vi "E2E Save Instrument.vi"() -> ()   [LabVIEW 2026]
panel:
  out "error out":errorcluster
  in  "vi path":path
  in  "Path to Saved File":path
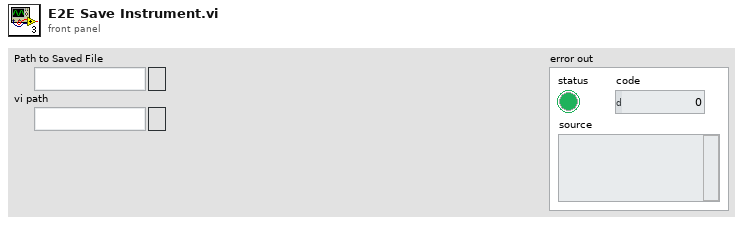
[diagram p1: front panel]
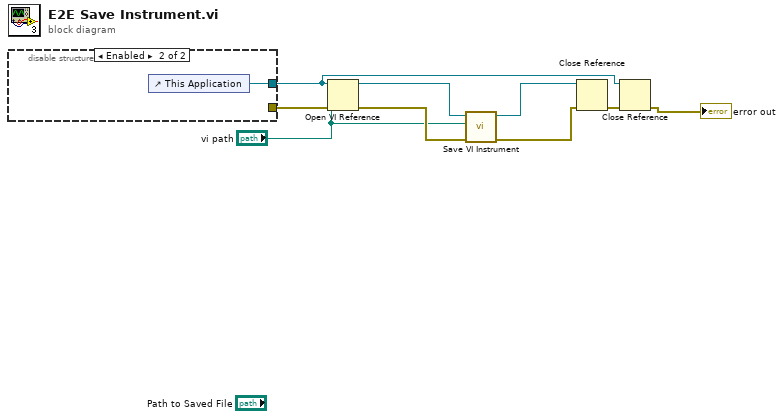
[diagram p0: block diagram]
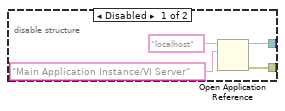
[diagram p2: hidden frame]
diagram:
  n1 = disable-structure shown="Enabled" {
    disable-tunnel: [w13 _] -> w9
    disable-tunnel: [w12 w14] -> w6
    frame Disabled {
      n2 = Open Application Reference(10:"Main Application Instance/VI Server" ("machine name (\"\":  open local reference)"), 11:"localhost" ("machine name (\"\":  open local reference)")) -> (0:w13:errorcluster, 3:w12:refnum<vi>)  [unwired: 2 in]
    }
    frame Enabled {
      n3 = control-ref of="This Application"() -> (w14:refnum<vi>)
    }
  }
  n4 = Open VI Reference(application reference (local)=w6, vi path="vi path", error in (no error)=w9) -> (vi reference=w5:refnum<vi>, error out=w8:errorcluster)  [unwired: 3 in]
  n5 = call "Save VI Instrument.vi"("error in (no error)"=w8, "vi path"="vi path", "VI in"=w5) -> ("error out"=w3:errorcluster, "VI out"=w4:refnum<vi>)  [unwired: 7 in]
  n6 = Close Reference(reference=w4, error in (no error)=w3) -> (error out=w7:errorcluster)
  n7 = Close Reference(reference=w6, error in (no error)=w7) -> (error out=→"error out":errorcluster)
